vi "Open App Ref.vi"(8 "error in (no error)":errorcluster, 11 "Editor in":refnum<class "Editor.lvclass">) -> (0 "error out":errorcluster, 3 "Editor out":refnum<class "Editor.lvclass">)   [LabVIEW 2020, in "VolatusGUIEditor.lvlib" / "Editor.lvclass"]
uses:
  Editor.lvclass
  Editor.lvclass/Editor.ctl
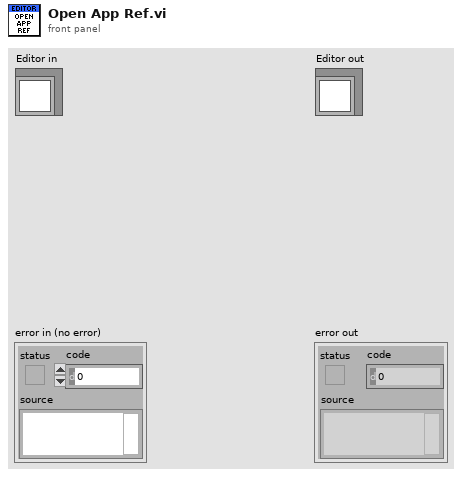
[diagram p1: front panel]
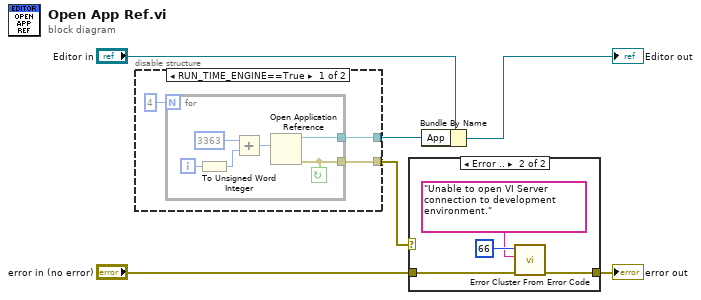
[diagram p0: block diagram]
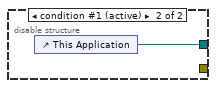
[diagram p2: hidden frame]
diagram:
  n1 = disable-structure shown="RUN_TIME_ENGINE==True" {
    disable-tunnel: [w9 w16] -> w4
    disable-tunnel: [w7 _] -> w2
    frame condition #0 {
      n2 = for {
        N: 4 -> [_]
        tunnel: [w14] -> w9
        tunnel: [w10] -> w7
        i -> [w12]
        stop <- w10 continue-if-true
        n3 = To Unsigned Word Integer(number=w12) -> (unsigned 16bit integer=w11:u16)
        n4 = Add(x=u16 3363 ("port number or service name (3363)"), y=w11) -> (x+y=w13:u16)
        n5 = Open Application Reference(10:w13) -> (0:w10:errorcluster, 3:w14:refnum<vi>)  [unwired: 3 in]
      }
    }
    frame condition #1 (active) {
      n6 = control-ref of="This Application"() -> (w16:refnum<vi>)
    }
  }
  n7 = case shown="Error .." w2 {
    tunnel: "error in (no error)" -> [w17 w20]
    tunnel: [w17 w21] -> w1
    frame No Error {
    }
    frame Error {
      n8 = call <vilib>:"Error Cluster From Error Code.vi"("error in (no error)"=w20, "error message (\"\")"="Unable to open VI Server connection to development environment.", "error code (0)"=66) -> ("error out"=w21:errorcluster)  [unwired: 6 in]
    }
  }
  "error out" <- w1
  n9 = Bundle By Name(cluster="Editor in", "App"=w4) -> (→"Editor out":refnum<class "Editor.lvclass">)
